vi "Configure Input POW TRAN ABOperation.vi"(6 "B Width (1)":dbl=1.0 min=0.0 max=120.0 step=1.0 format="%#.3f", 7 "A Width (1)":dbl=1.0 min=0.0 max=120.0 step=1.0 format="%#.3f", 8 "error in (no error)":errorcluster, 9 "B Level Value (2)":dbl=2.0 min=0.0 max=7500.0 step=1.0 format="%.3f", 10 "A Level Value (1)":dbl=1.0 min=0.0 max=7500.0 step=1.0 format="%.3f", 11 "VISA resource name":refnum<visa-resource-name>) -> (0 "error out":errorcluster, 3 "VISA resource name out":refnum<visa-resource-name>)   [LabVIEW 2015, in "IT8900A-E.lvlib"]
doc: "The command specifies that the switching value of the input power transient generator switches between ab values.And the switching pulse width of the input power."
uses:
  <instrlib>/IT8900/IT8900A-E.lvlib
panel:
  # "s"
  # "s"
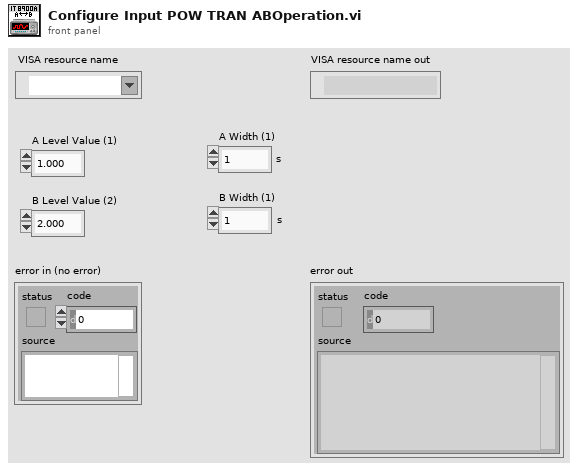
[diagram p1: front panel]
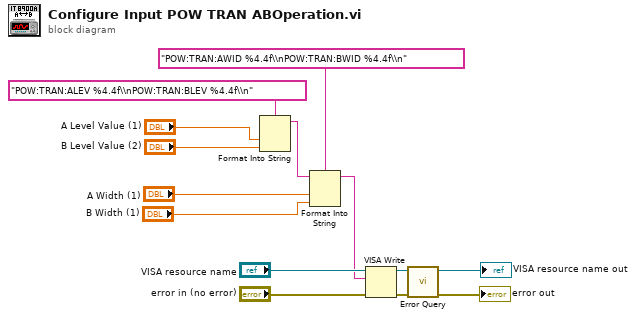
[diagram p0: block diagram]
diagram:
  n1 = Format Into String(format string="POW:TRAN:ALEV %4.4f\\nPOW:TRAN:BLEV %4.4f\\n", "A Level Value (1)", "B Level Value (2)") -> (resulting string=w3:string)  [unwired: 2 in, 1 out]
  n2 = Format Into String(format string="POW:TRAN:AWID %4.4f\\nPOW:TRAN:BWID %4.4f\\n", initial string=w3, "A Width (1)", "B Width (1)") -> (resulting string=w1:string)  [unwired: 1 in, 1 out]
  n3 = VISA Write(VISA resource name="VISA resource name", write buffer=w1, error in (no error)="error in (no error)") -> (VISA resource name out=w11:refnum<visa-resource-name>, error out=w12:errorcluster)  [unwired: 1 out]
  n4 = call <instrlib>:"Error Query.vi"("error in (no error)"=w12, "VISA resource name"=w11) -> ("error out"=→"error out":errorcluster, "VISA resource name out"=→"VISA resource name out":refnum<visa-resource-name>)  [unwired: 6 in, 2 out]
